vi "Check In Tolerance.vi"(0 "Model in":refnum<class "Model.lvclass">, 5 "Expected":dbl, 7 "Tolerance":dbl, 9 "Actual":dbl, 11 "error in (no error)":errorcluster) -> (4 "Model out":refnum<class "Model.lvclass">, 6 "Pass":bool, 15 "error out":errorcluster)   [LabVIEW 2016]
uses:
  Model.lvclass
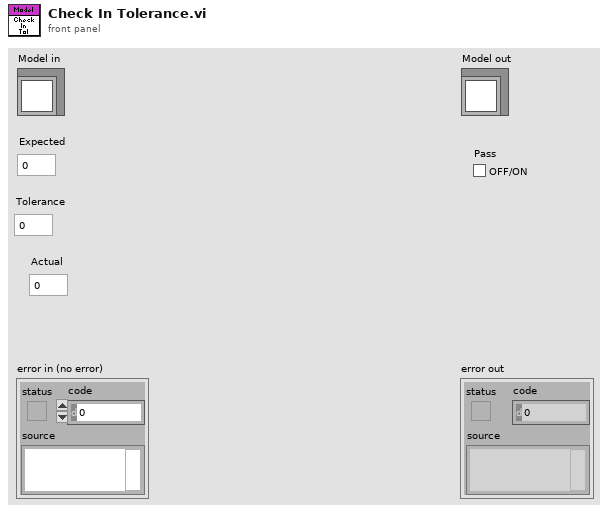
[diagram p1: front panel]
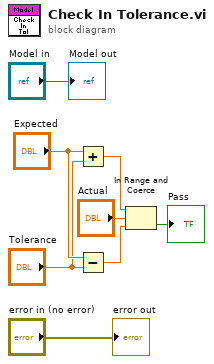
[diagram p0: block diagram]
diagram:
  n1 = Add(x="Expected", y="Tolerance") -> (x+y=w5:dbl)
  n2 = Subtract(x="Expected", y="Tolerance") -> (x-y=w4:dbl)
  n3 = In Range and Coerce(upper limit=w5, x="Actual", lower limit=w4) -> (In Range?=→"Pass":bool)  [unwired: 1 out]
  "error out" <- "error in (no error)"
  "Model out" <- "Model in"
